vi "Snow.vi"() -> ()   [LabVIEW 2019]
doc: "Just small demo - how to \"animate\" image with cyclical change of the palette.\nLabVIEW code - Andrey Dmitriev (2012-2019).\nArtwork: Mark J. Ferrari (http://www.markferrari.com/)"
uses:
  <vilib>/picture/picture.llb/imagedata.ctl
panel:
  in  "Stop Button":bool
  out "2D Picture":picture
  # "Artwork: Mark J. Ferrari (http://www.markferrari.com/)"
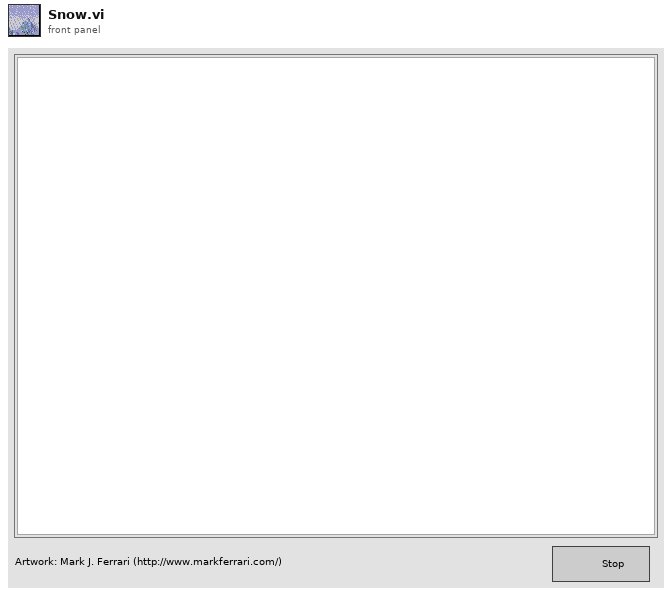
[diagram p1: front panel]
types:
  T1 = typedef "imagedata.ctl" = cluster{"image type":i32, "image depth":i32, "image":u8[], "mask":u8[], "colors":u32[], "Rectangle":cluster{"left":i16, "top":i16, "right":i16, "bottom":i16}}
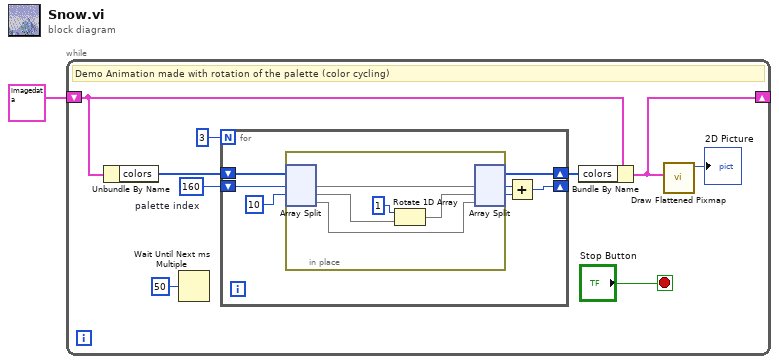
[diagram p0: block diagram]
diagram:
  n1 = while {
    shift-right: [w5] -> _
    shift-left: T1 {"image type"=0, "image depth"=8, "image"=array[307200 elements], "mask"=[], "colors"=[0, 12762850, 12499678, 12236510, 11974362, 11711194, 11448022, 11446998, 11184854, 10855894, 10330578, 10067406, 9804234, 9278922, 9015750, 8752578, 8489406, 8227262, 13292287, 9805270, 9016782, 8489410, 7700922, 7174578, 6648234, 6121889, 5595545, 5003665, 5267865, 5859745, 6123946, 6650294, 4216193, 8488382, 2636901, 11186918, 1845320, 7961002, 7434657, 7171485, 6646169, 6381969, 5856653, 5593481, 5856653, 6119825, 6382997, 6646169, 10068450, 9278918, 7699886, 3687549, 6385061, 3162213, 3163225, 11451110, 11451110, 11451110, 2105416, 8244, 265232, 1846348, 11982591, 9542090, 9802162, 6118797, 3424361, 13291250, 3158096, 4997209, 13291250, 7169409, 13291250, 65413, 16777215, 9803214, 5590129, 9248, 6152, 3072, 2048, 1024, 1024, 14344959, 6645097, 3414068, 262144, 3679292, 16777215, 11972338, 11316, 7200, 3084, 0, 0, 16711918, 2118984, 11284, 8196, 5120, 2048, 0, 0, 16711918, 9538957, 7959925, 5855577, 4998212, 3681324, 2365464, 1050632, 3682372, 7162956, 4730928, 3153944, 1050628, 0, 787460, 2627596, 3679256, 4730920, 6111288, 3679264, 1838092, 262144, 0, 0, 1839120, 3417124, 13291250, 10323357, 13291250, 11452130, 8221089, 13291250, 1842240, 9537974, 6381953, 3157056, 3682384, 2368592, 2368592, 2368592, 2368592, 13291250, 16185087, 14870271, 12502754, 11186898, 10068418, 8753590, 7963050, 6122905, 4477049, 3162209, 11449050, 10593746, 9804238, 9015750, 8489410, 2101264, 2101264, 2101264, 12502754, 2101264, 2101264, 2101264, 2101264, 2101264, 2101264, 4474973, 4474973, 4474973, 12502754, 4474973, 4474973, 4474973, 4474973, 4474973, 4474973, 7963050, 7963050, 7963050, 12502754, 7963050, 7963050, 7963050, 7963050, 7963050, 7963050, 9278906, 9278906, 9278906, 12502754, 9278906, 9278906, 9278906, 9278906, 9278906, 9278906, 10595026, 10595026, 10595026, 12502754, 10595026, 10595026, 10595026, 10595026, 10595026, 10595026, 12501730, 12501730, 12501730, 13818610, 12501730, 12501730, 12501730, 12501730, 12501730, 12501730, 16777215, 16777215, 16777215, 16777215, 16711918, 16711918, 16711918, 16711918, 16711918, 16711918, 16711918, 16711918, 16711918, 16711918, 16711918, 16711918, 16711918, 16711918, 16711918, 16711918, 16711918, 16711918, 16711918, 16711918, 16711918, 16711918, 16711918, 16711918, 16741632, 5046016, 262399, 16711684, 16772608, 16711918, 10611455, 16777215], "Rectangle"={"left"=0, "top"=0, "right"=640, "bottom"=480}} ("image data") -> [w9]
    stop <- "Stop Button" stop-if-true
    w2 = 160  # palette index
    # "Demo Animation made with rotation of the palette (color cycling)"
    n2 = Unbundle By Name(w9) -> ("colors"=w10:u32[])
    n3 = Wait Until Next ms Multiple(millisecond multiple=u32 50 ("milliseconds to wait")) -> ()  [unwired: 1 out]
    n4 = for {
      N: 3 -> [_]
      shift-right: [w15] -> w4
      shift-left: w10 -> [w17]
      shift-right: [w14] -> _
      shift-left: w2 -> [w16]
      n5 = in-place {
        n6 = in-place-split #1(w17, w16, 10) -> (w20:u32[], w22:u32[], w19:u32[])
        n7 = Rotate 1D Array(1:w22, 2:1 ("n")) -> (0:w21:u32[])
        n8 = in-place-split #1(w20, w21, w19) -> (w15:u32[], w13:i32, w12:i32)
      }
      n9 = Add(x=w13, y=w12) -> (x+y=w14:i32)
    }
    n10 = Bundle By Name(cluster=w9, "colors"=w4) -> (w5:T1)
    n11 = call <vilib>:"Draw Flattened Pixmap.vi"("image data"=w5) -> ("new picture"=→"2D Picture":picture)  [unwired: 8 in]
  }
